vi "Test_Observe_ModelPublication_OK.vi"(8 "error in (no error)":errorcluster, 11 "TestObservation In":refnum<class "TestPubSubRouting.lvclass">) -> (0 "error out":errorcluster, 3 "TestObservation Out":refnum<class "TestPubSubRouting.lvclass">)   [LabVIEW 2017, in "TestPubSubRouting.lvlib" / "TestPubSubRouting.lvclass"]
uses:
  TestPubSubRouting.lvclass
  gpm_packages/@cs/mva-core/Source/Mediator/Mediator/Mediator.lvclass
  <vilib>/ActorFramework/Actor/Actor.lvclass
  ObservingViewable/ObservingViewable.lvclass
  <vilib>/ActorFramework/Stop Msg/Stop Msg.lvclass
  PublishingModel/PublishingModel.lvclass
  ObservingViewModel/ObservingViewModel.lvclass
  be72e04e-1098-4f6e-bc5d-93c8d08dbeb7.vi
  C:/Program Files (x86)/National Instruments/LabVIEW 2017/vi.lib/ActorFramework/Actor/Actor.lvclass
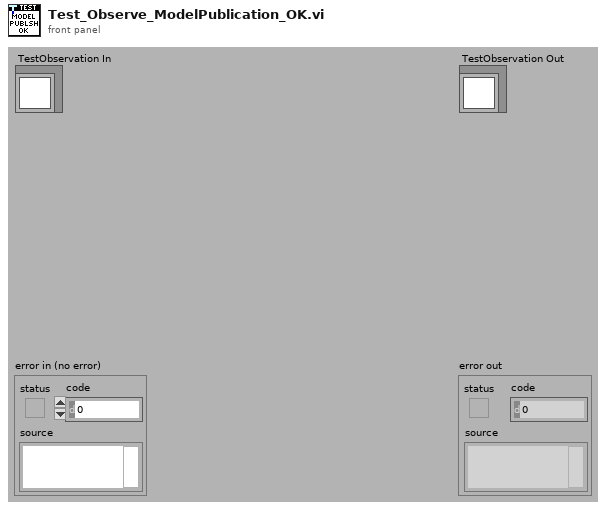
[diagram p1: front panel]
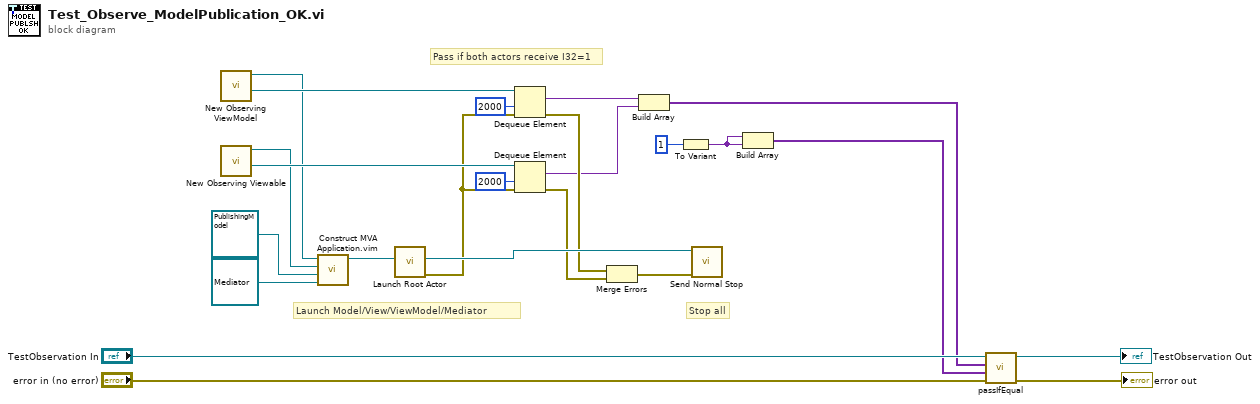
[diagram p0: block diagram]
diagram:
  # "Stop all"
  # "Launch Model/View/ViewModel/Mediator"
  # "Pass if both actors receive I32=1"
  n1 = call "New Observing ViewModel.vi"() -> ("Test Reply Queue"=w11:refnum<queue>, "ObservingViewModel Out"=w2:refnum<class "ObservingViewModel.lvclass">)  [unwired: 10 in]
  n2 = call "New Observing Viewable.vi"() -> ("Test Reply Queue"=w17:refnum<queue>, "ObservingViewable out"=w3:refnum<class "ObservingViewable.lvclass">)  [unwired: 10 in]
  n3 = call "Construct MVA Application.vim"("Mediator Type"=refnum<class "Mediator.lvclass"> refnum ("Mediator.lvlib:Mediator.lvclass"), "Model Type"=refnum<class "PublishingModel.lvclass"> refnum ("PublishingModel.lvclass"), "Startup View Configuration"=w3, "IViewModel In"=w2) -> ("IViewModel Out"=w18:refnum<class "ObservingViewModel.lvclass">)  [unwired: 7 in]
  n4 = call <vilib>:"Launch Root Actor.vi"("Actor"=w18) -> ("error out"=w1:errorcluster, "Actor's Enqueuer"=w15:refnum<class "Message Enqueuer.lvclass">)  [unwired: 9 in]
  n5 = Dequeue Element(queue=w11, timeout in ms (-1)=2000, error in (no error)=w1) -> (element=w8:variant, error out=w9:errorcluster)  [unwired: 2 out]
  n6 = Dequeue Element(queue=w17, timeout in ms (-1)=2000, error in (no error)=w1) -> (element=w7:variant, error out=w14:errorcluster)  [unwired: 2 out]
  n7 = Merge Errors(w9, w14) -> (w10:errorcluster)
  n8 = Build Array(w8, w7) -> (w6:variant[])
  n9 = To Variant(anything=1) -> (Variant=w4:variant)
  n10 = call <vilib>:"Send Normal Stop.vi"("error in (no error)"=w10, "Message Enqueuer"=w15) -> ()  [unwired: 9 in, 1 out]
  n11 = Build Array(w4, w4) -> (w5:variant[])
  n12 = call-dynamic "passIfEqual.vi"("error in (no error)"="error in (no error)", "y"=w5, "x"=w6, "TestCase in"="TestObservation In") -> ("error out"=→"error out":errorcluster, "TestCase out"=→"TestObservation Out":refnum<class "TestPubSubRouting.lvclass">)  [unwired: 6 in]
